vi "xiC - IMAQ - Play_ValChange.vi"(8 "error in (no error)":errorcluster, 11 "Attributes In":T1) -> (0 "error out":errorcluster, 3 "Attributes Out":T1)   [LabVIEW 2018]
uses:
  xiC - IMAQ - Attributes.ctl
  D:/codes labview/VisionLibrariesXimea/xiLib/xiLIB_64bit/xiLIB/xiCamLib/API/x64/xiApi.NETX64.dll
  xiCamLib/API/x64/xiApi.NETX64.dll
  xiC - IMAQ - TreeDisplayType.ctl
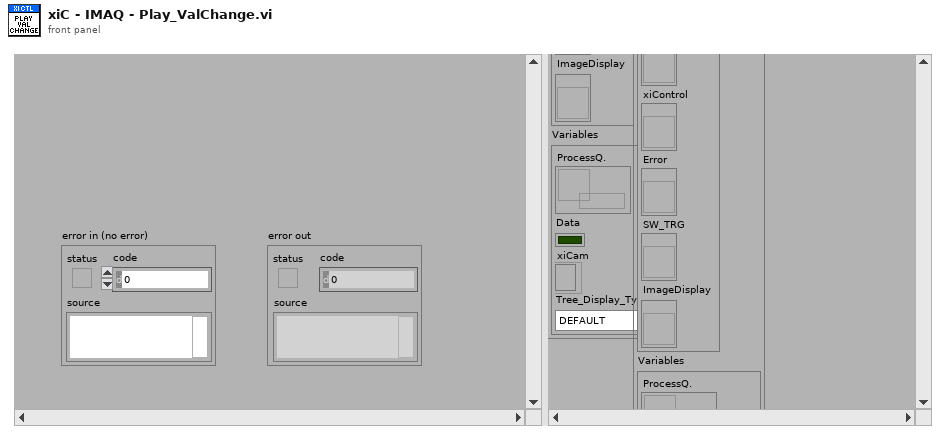
[diagram p1: front panel]
types:
  T1 = typedef "xiC - IMAQ - Attributes.ctl" = cluster{"Controls":cluster{"VI Ref.":refnum<vi>, "Tree":refnum<vi>, "Info":refnum<vi>, "PRMName":refnum<vi>, "xiControl":refnum<vi>, "Error":refnum<vi>, "SW_TRG":refnum<vi>, "ImageDisplay":refnum<vi>}, "Variables":cluster{"ProcessQ.":refnum<queue>, "Data":bool, "xiCam":refnum<k24>, "Tree_Display_Type":T2}}
  T2 = typedef "xiC - IMAQ - TreeDisplayType.ctl" = enum16{"DEFAULT", "HIDE_MAX_MIN"}
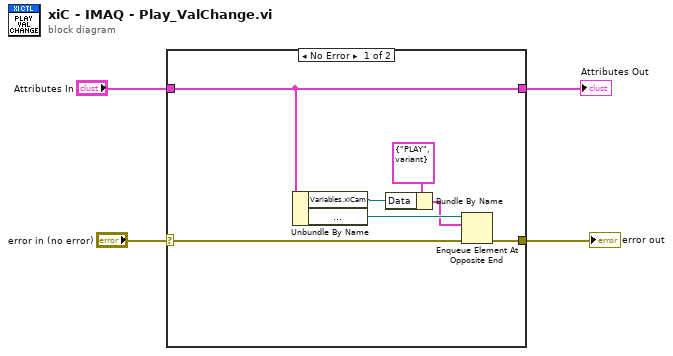
[diagram p0: block diagram]
diagram:
  n1 = case shown="No Error" "error in (no error)" {
    selector: "error in (no error)" -> [w6 w13]
    tunnel: [w5 w13] -> w3
    tunnel: "Attributes In" -> [w10 w12]
    tunnel: [w10 w12] -> w1
    frame No Error {
      n2 = Unbundle By Name(w10) -> ("Variables.xiCam"=w8:refnum<k24>, "Variables.ProcessQ."=w11:refnum<queue>)
      n3 = Bundle By Name(cluster=cluster{"State":string, "Data":variant} {"State"="PLAY", "Data"=variant} ("element"), "Data"=w8) -> (w7:cluster{"State":string, "Data":variant})
      n4 = Enqueue Element At Opposite End(queue=w11, element=w7, error in (no error)=w6) -> (error out=w5:errorcluster)  [unwired: 1 in, 2 out]
    }
    frame Error {
    }
  }
  "error out" <- w3
  "Attributes Out" <- w1
